vi "for loop.vi"() -> ()   [LabVIEW 2020]
panel:
  out "Waveform Chart":i32(graph)
  out "Numeric 3":dbl
  out "Numeric 2":u32
  in  "Numeric":u32
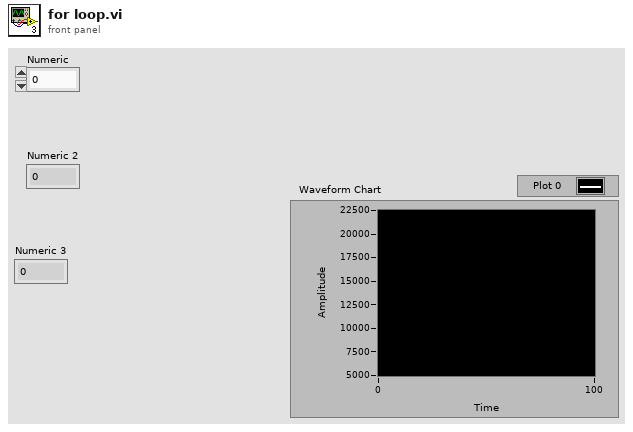
[diagram p1: front panel]
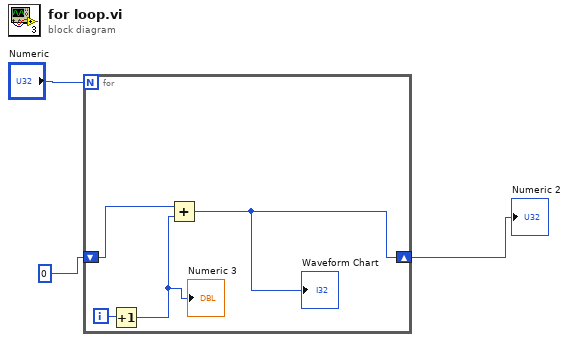
[diagram p0: block diagram]
diagram:
  n1 = for {
    N: "Numeric" -> [_]
    shift-right: [w4] -> w1
    shift-left: 0 -> [w6]
    i -> [w7]
    n2 = Increment(x=w7) -> (x+1=w5:i32)
    "Numeric 3" <- w5
    n3 = Add(x=w6, y=w5) -> (x+y=w4:i32)
    "Waveform Chart" <- w4
  }
  "Numeric 2" <- w1
